vi "Dropdown - Init Case.vi"(11 "Unit Abbreviations":string[](array[string])) -> (0 "Error Out":errorcluster)   [LabVIEW 2013]
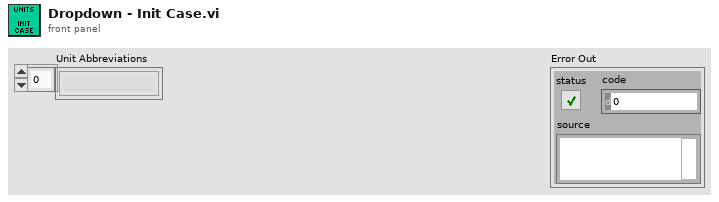
[diagram p1: front panel]
types:
  T1 = enum16{"Set Abbreviations", "Set Engine Mode", "Set Enum Position", "Get Abbreviation", "Write Abbreviation", "Read Enum Position", "Read Engine Mode", "Read Abbreviations", "Engine Started", "Check Engine", "Init Global", "Set Cursor", "Read Cursor"}
  T2 = enum16{"Idle", "Reveal Dropdown", "Hide FP", "Set Options"}
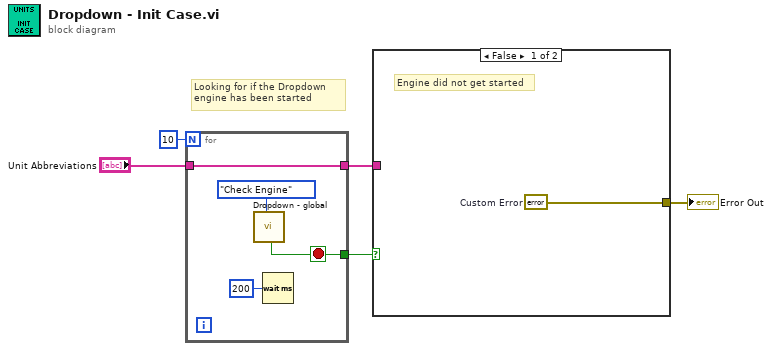
[diagram p0: block diagram]
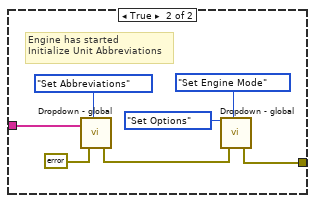
[diagram p2: hidden frame]
diagram:
  # "Looking for if the Dropdown\nengine has been started"
  n1 = for {
    N: 10 -> [_]
    tunnel: "Unit Abbreviations" -> [w9]
    tunnel: [w9] -> w3
    tunnel: [w7] -> w5
    stop <- w7 stop-if-true
    n2 = call "Dropdown - global.vi"("Global Mode"=T1."Check Engine") -> ("Engine Started"=w7:bool)  [unwired: 10 in, 8 out]
    n3 = Wait (ms)(milliseconds to wait=u32 200) -> ()  [unwired: 1 out]
  }
  n4 = case shown="False" w5 {
    tunnel: w3 -> [_ w15]
    tunnel: [w10 w11] -> w1
    frame False {
      w10 = errorcluster {"status"=TRUE, "code"=0, "source"="Custom Error: The dropdown engine was not started"}  # Custom Error
      # "Engine did not get started"
    }
    frame True {
      # "Engine has started\nInitialize Unit Abbreviations"
      n5 = call "Dropdown - global.vi"("AbbrS In"=w15, "Error In"=errorcluster {"status"=FALSE, "code"=0, "source"=""} ("error constant"), "Global Mode"=T1."Set Abbreviations") -> ("Error Out"=w17:errorcluster)  [unwired: 8 in, 8 out]
      n6 = call "Dropdown - global.vi"("Engine Mode In"=T2."Set Options", "Error In"=w17, "Global Mode"=T1."Set Engine Mode") -> ("Error Out"=w11:errorcluster)  [unwired: 8 in, 8 out]
    }
  }
  "Error Out" <- w1
